vi "Strip Cluster.vi"(6 "Configuration":T1, 7 "Prefix Name":string, 8 "error in (no error)":errorcluster, 9 "Values in":string[](array[string]), 10 "Key in":string[](array[string]), 11 "Cluster Refnum":refnum<vi>) -> (0 "error out":errorcluster, 1 "Values":string[](array[string]), 2 "Keys":string[](array[string]), 3 "Cluster Refnum (Dup)":refnum<vi>)   [LabVIEW 2019]
doc: "Wire any cluster control reference to this VI. The VI will generate keys and values for each element of the cluster. The operation is recursive, so keys will be generated for array and cluster elements as well. The key and value inputs are required to support recursion, but may be used to chain the outputs of multiple strip operations over several clusters.\n\nSupported data types, as of 12/20/06:\nBoolean (TRUE if value is <> 0 or <> \"FALSE\")\nPath\nDouble\nString\nEnumerated Type (value can be an integer or enum string)\nTime stamp (value saved as a double)\nArray (recursive)\nCluster (recursive)\nShared Variable Reference\nRing Control (value can be an integer or string)\nVISA resource name\nCombo Box (value can be the string or combo box value)\n\nKey format:\n<prefix>.<control name_1>[.M.<control name_2>]...[.<control name_N>]\n\nIf the <prefix> input is an empty string, the label of the input cluster will be used instead.\n\n<control name> is the name of a control in the cluster. The control may be any supported type, including arrays and clusters.\n\n<control name_N>.n.<control name_N+1> is the Mth element of the <control name_N> array, where the array element is named <control name_N+1>. The array element name is not optional."
uses:
  Cluster Formatting.ctl
panel:
  in  "Strip Cluster":refnum<vi>
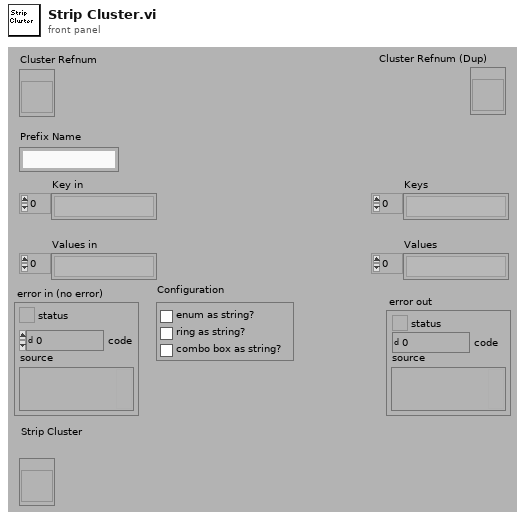
[diagram p1: front panel]
types:
  T1 = typedef "Cluster Formatting.ctl" = cluster{"enum as string?":bool, "ring as string?":bool, "combo box as string?":bool}
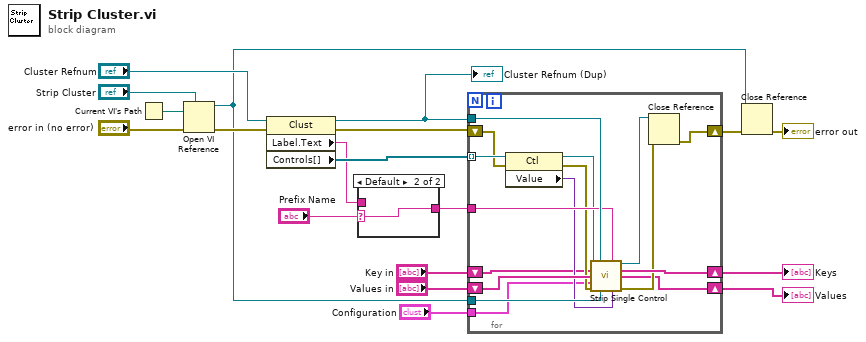
[diagram p0: block diagram]
diagram:
  n1 = Current VI's Path() -> (path=w16:path)
  n2 = Open VI Reference(type specifier VI Refnum (for type only)="Strip Cluster", vi path=w16, error in (no error)="error in (no error)") -> (vi reference=w3:refnum<vi>, error out=w14:errorcluster)  [unwired: 3 in]
  n3 = property class="Clust"(reference="Cluster Refnum", error in=w14) -> (reference out=w12:refnum<vi>, error out=w19:errorcluster, "Label.Text"=w5:string, "Controls[]"=w18:refnum<vi>[])
  "Cluster Refnum (Dup)" <- w12
  n4 = case shown="Default" "Prefix Name" {
    selector: "Prefix Name" -> [_ w21]
    tunnel: w5 -> [w20 _]
    tunnel: [w20 w21] -> w7
    frame "" {
    }
    frame Default {
    }
  }
  n5 = for {
    tunnel: w18 -> [w32] mode=indexing
    shift-right: [w25] -> w4
    shift-left: w19 -> [w29]
    tunnel: w3 -> [w37]
    tunnel: w12 -> [w36]
    shift-right: [w22] -> w8
    shift-left: "Values in" -> [w35]
    shift-right: [w34] -> w9
    shift-left: "Key in" -> [w24]
    tunnel: w7 -> [w33]
    tunnel: "Configuration" -> [w23]
    n6 = property class="Ctl"(reference=w32, error in=w29) -> (reference out=w31:refnum<vi>, error out=w28:errorcluster, "Value"=w30:variant)
    n7 = call "Strip Single Control.vi"("Ctl Refnum"=w31, "Cluster Refnum"=w36, "Label.Text"=w33, "Keys in"=w24, "Values in"=w35, "Formatting"=w23, "error in (no error)"=w28, "Strip Cluster"=w37, "Value"=w30) -> ("Ctl Refnum"=w27:refnum<vi>, "Keys out"=w34:string[], "Values out"=w22:string[], "error out"=w26:errorcluster)  [unwired: 3 in]
    n8 = Close Reference(reference=w27, error in (no error)=w26) -> (error out=w25:errorcluster)
  }
  "Keys" <- w9
  "Values" <- w8
  n9 = Close Reference(reference=w3, error in (no error)=w4) -> (error out=→"error out":errorcluster)
